vi "Parameters_Request.vi"(8 "error in (no error)":errorcluster, 10 "Active Channels":u16[](array[numeric]), 11 "VISA resource name":refnum<visa-resource-name>="Master_Oscilloscope") -> (0 "error out":errorcluster, 1 "Parameters(array)":string[](array[string]), 3 "VISA resource name out":refnum<visa-resource-name>)   [LabVIEW 2020]
panel:
  # "PARAMETERS REQUEST"
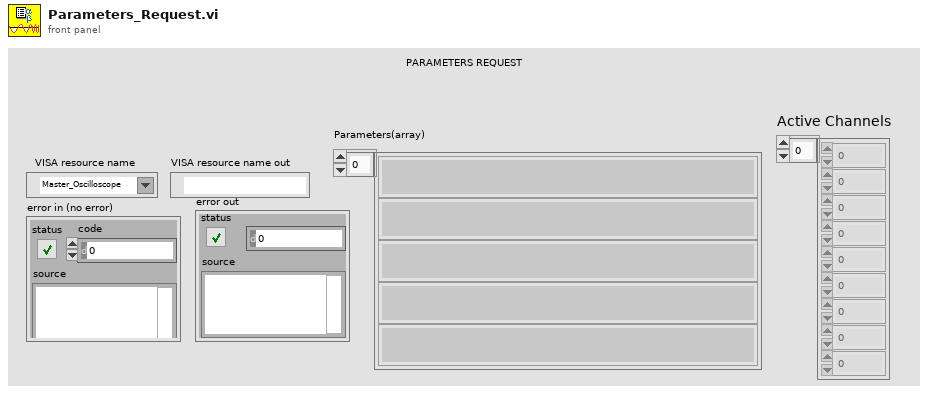
[diagram p1: front panel]
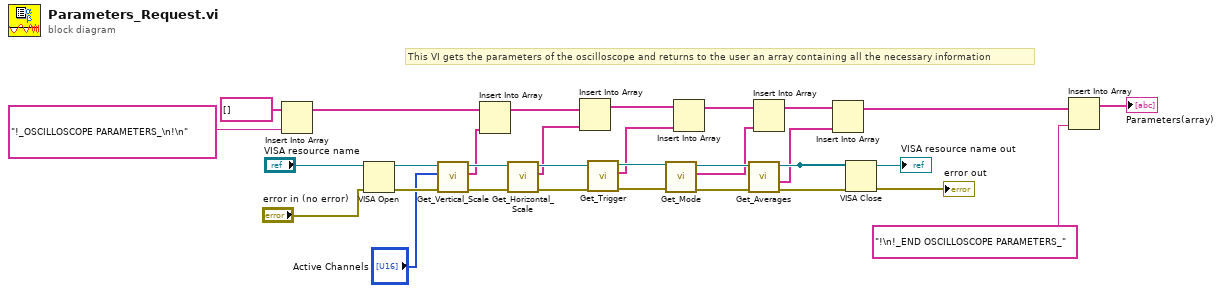
[diagram p0: block diagram]
diagram:
  # "This VI gets the parameters of the oscilloscope and returns to the user an array containing all the necessary information"
  n1 = Insert Into Array(array=string[] [], new element="!_OSCILLOSCOPE PARAMETERS_\n!\n") -> (w6:string[])  [unwired: 1 in]
  n2 = VISA Open(error in (no error)="error in (no error)", VISA resource name="VISA resource name") -> (VISA resource name=w29:refnum<visa-resource-name>, error out=w28:errorcluster)  [unwired: 3 in]
  n3 = call "Get_Vertical_Scale.vi"("error in (no error)"=w28, "Active_Channels"="Active Channels", "VISA resource name"=w29) -> ("error out"=w25:errorcluster, "Vertical_Parameters"=w5:string[], "VISA resource name out"=w26:refnum<visa-resource-name>)  [unwired: 5 in]
  n4 = Insert Into Array(array=w6, new element=w5) -> (w4:string[])  [unwired: 1 in]
  n5 = call "Get_Horizontal_Scale.vi"("error in (no error)"=w25, "VISA resource name"=w26) -> ("error out"=w23:errorcluster, "Horizontal_Parameters"=w15:string[], "VISA resource name out"=w24:refnum<visa-resource-name>)  [unwired: 6 in]
  n6 = Insert Into Array(array=w4, new element=w15) -> (w14:string[])  [unwired: 1 in]
  n7 = call "Get_Trigger.vi"("error in (no error)"=w23, "VISA resource name"=w24) -> ("error out"=w21:errorcluster, "Trigger_Parameters"=w13:string[], "VISA resource name out"=w22:refnum<visa-resource-name>)  [unwired: 7 in]
  n8 = call "Get_Mode.vi"("error in (no error)"=w21, "VISA resource name"=w22) -> ("error out"=w19:errorcluster, "Mode"=w11:string[], "VISA resource name out"=w20:refnum<visa-resource-name>)  [unwired: 5 in]
  n9 = Insert Into Array(array=w14, new element=w13) -> (w12:string[])  [unwired: 1 in]
  n10 = call "Get_Averages.vi"("error in (no error)"=w19, "VISA resource name"=w20) -> ("error out"=w17:errorcluster, "Averages"=w9:string[], "VISA resource name out"=w18:refnum<visa-resource-name>)  [unwired: 6 in, 1 out]
  "VISA resource name out" <- w18
  n11 = Insert Into Array(array=w12, new element=w11) -> (w10:string[])  [unwired: 1 in]
  n12 = Insert Into Array(array=w10, new element=w9) -> (w3:string[])  [unwired: 1 in]
  n13 = VISA Close(VISA resource name=w18, error in (no error)=w17) -> (error out=→"error out":errorcluster)
  n14 = Insert Into Array(array=w3, new element="!\n!_END OSCILLOSCOPE PARAMETERS_" ("new element/subarray")) -> (→"Parameters(array)":string[])  [unwired: 1 in]
